vi "roi_mean.vi"(7 "aal":path=path "C:/AeroFS/Working/Voxel-wise connectivity/NIfTI-1 Data/Data/AAL_61x73x61_YCG.nii", 11 "file (use dialog)":path) -> ()   [LabVIEW 2014]
uses:
  variant_3d.vi
  <vilib>/Utility/file.llb/Write To Spreadsheet File (DBL).vi
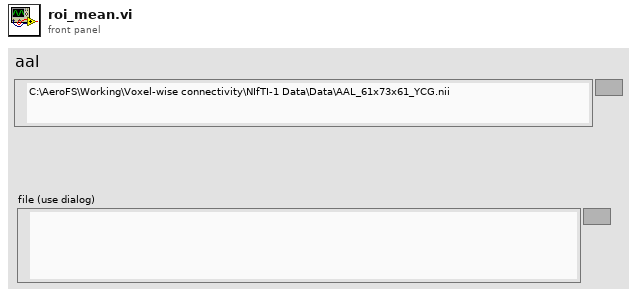
[diagram p1: front panel]
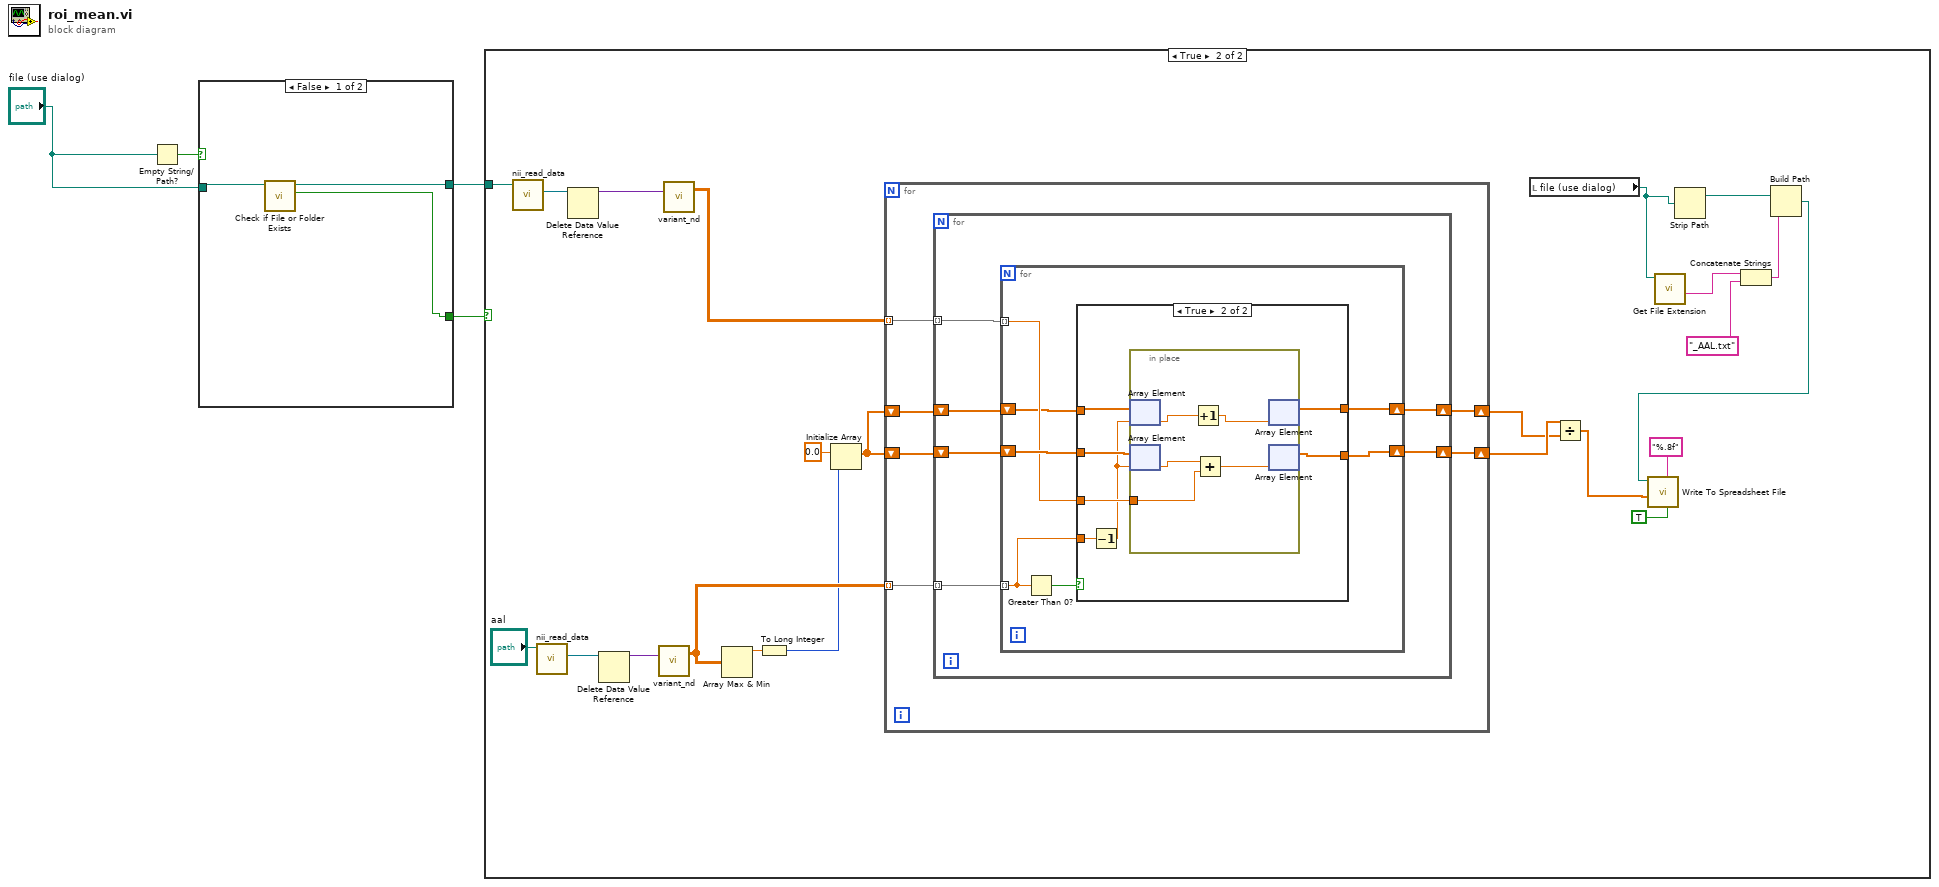
[diagram p0: block diagram]
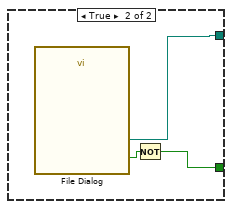
[diagram p4: hidden frame]
diagram:
  n1 = Empty String/Path?(string/path="file (use dialog)") -> (empty?=w4:bool)
  n2 = case shown="False" w4 {
    tunnel: "file (use dialog)" -> [w7 _]
    tunnel: [w5 w10] -> w2
    tunnel: [w6 w8] -> w1
    frame False {
      n3 = call <vilib>:"Check if File or Folder Exists.vi"("path"=w7) -> ("file or folder exists?"=w5:bool, "dup path"=w6:path)  [unwired: 8 in, 1 out]
    }
    frame True {
      n4 = call "File Dialog"() -> ("selected path"=w8:path, "cancelled"=w9:bool)  [unwired: 12 in, 2 out]
      n5 = Not(x=w9) -> (.not. x?=w10:bool)
    }
  }
  n6 = case shown="True" w2 {
    tunnel: w1 -> [_ w33]
    frame False {
    }
    frame True {
      n7 = call "nii_read_data.vi"("file (use dialog)"=w33) -> ("data value reference"=w32:refnum<data-value>)  [unwired: 6 in, 4 out]
      n8 = call "nii_read_data.vi"("file (use dialog)"="aal") -> ("data value reference"=w31:refnum<data-value>)  [unwired: 6 in, 4 out]
      n9 = Delete Data Value Reference(data value reference=w32) -> (data value=w11:variant)  [unwired: 1 in, 1 out]
      n10 = Delete Data Value Reference(data value reference=w31) -> (data value=w12:variant)  [unwired: 1 in, 1 out]
      n11 = call-poly "variant_nd.vi"("variant"=w12) -> ("data"=w28:sgl[][][])  [unwired: 2 in]
      n12 = call-poly "variant_nd.vi"("variant"=w11) -> ("data"=w29:sgl[][][])  [unwired: 2 in]
      n13 = Array Max & Min(array=w28) -> (max value=w27:sgl)  [unwired: 3 out]
      n14 = To Long Integer(number=w27) -> (32bit integer=w13:i32)
      n15 = Initialize Array(0.0 ("element"), w13) -> (w25:dbl[])
      n16 = for {
        tunnel: w28 -> [w39] mode=indexing
        tunnel: w29 -> [w38] mode=indexing
        shift-right: [w36] -> w24
        shift-left: w25 -> [w37]
        shift-right: [w35] -> w23
        shift-left: w25 -> [w34]
        n17 = for {
          tunnel: w39 -> [w45] mode=indexing
          tunnel: w38 -> [w44] mode=indexing
          shift-right: [w42] -> w36
          shift-left: w37 -> [w43]
          shift-right: [w41] -> w35
          shift-left: w34 -> [w40]
          n18 = for {
            tunnel: w45 -> [w48] mode=indexing
            tunnel: w44 -> [w50] mode=indexing
            shift-right: [w49] -> w42
            shift-left: w43 -> [w51]
            shift-right: [w46] -> w41
            shift-left: w40 -> [w47]
            n19 = Greater Than 0?(x=w48) -> (x > 0?=w52:bool)
            n20 = case shown="True" w52 {
              tunnel: w51 -> [w54 w61]
              tunnel: w50 -> [_ w60]
              tunnel: [w54 w59] -> w49
              tunnel: w48 -> [_ w58]
              tunnel: w47 -> [w53 w57]
              tunnel: [w53 w55] -> w46
              frame False {
              }
              frame True {
                n21 = Decrement(x=w58) -> (x-1=w56:sgl)
                n22 = in-place {
                  in-place-border: w60 -> [w65]
                  n23 = in-place-array #1(w57, w56) -> (w63:dbl)
                  n24 = in-place-array #2(w61, w56) -> (w66:dbl)
                  n25 = Increment(x=w63) -> (x+1=w62:dbl)
                  n26 = Add(x=w66, y=w65) -> (x+y=w64:dbl)
                  n27 = in-place-array #1(w62) -> (w55:dbl[])  [unwired: 1 out]
                  n28 = in-place-array #2(w64) -> (w59:dbl[])  [unwired: 1 out]
                }
              }
            }
          }
        }
      }
      n29 = local read "file (use dialog)"() -> (w19:path)
      n30 = Divide(x=w24, y=w23) -> (x/y=w20:dbl[])
      n31 = call <vilib>:"Get File Extension.vi"("file"=w19) -> ("filename without extension"=w14:string)  [unwired: 7 in, 3 out]
      n32 = Strip Path(path=w19) -> (stripped path=w18:path)  [unwired: 1 out]
      n33 = Concatenate Strings(w14, "_AAL.txt" ("string")) -> (w16:string)
      n34 = Build Path(base path=w18, name or relative path=w16) -> (appended path=w15:path)
      n35 = call-poly <vilib>:"Write To Spreadsheet File.vi"("transpose? (no:F)"=TRUE, "format (%.3f)"="%.8f", "1D data"=w20, "file path (dialog if empty)"=w15) -> ()  [unwired: 4 in, 1 out]
    }
  }
